vi "Flatten.vi"(6 "Persistence in":refnum<class "IPersist.lvclass">, 7 "Linked List Ref":refnum<data-value>, 8 "error in (no error)":errorcluster, 9 "Indent":i32, 10 "Active Unique ID":string, 11 "Subsequence in":refnum<class "Subsequence.lvclass">) -> (0 "error out":errorcluster, 2 "Active Unique ID out":string, 3 "Flattened Test Executive":string[](array[string]), 4 "Persistence out":refnum<class "IPersist.lvclass">, 5 "Linked List Ref out":refnum<data-value>)   [LabVIEW 2019, in "Test Executive.lvlib" / "Subsequence.lvclass"]
uses:
  <vilib>/gpm_packages/@cs/test-executive/Source/Test Executive/Subsequence/Subsequence.lvclass
  <vilib>/gpm_packages/@cs/linked-list/Source/Linked List/ILinkedList/ILinked List.lvclass
  <vilib>/gpm_packages/@cs/persistence/source/IPersist/IPersist.lvclass
  <vilib>/gpm_packages/@cs/test-executive/Source/Test Executive/Executioner/Executioner.lvclass
  <vilib>/gpm_packages/@cs/linked-list/Source/Linked List/Linked List Ref/Linked List Ref.lvclass
  <vilib>/gpm_packages/@cs/linked-list/Source/String Manipulation/String Manipulation.lvlib
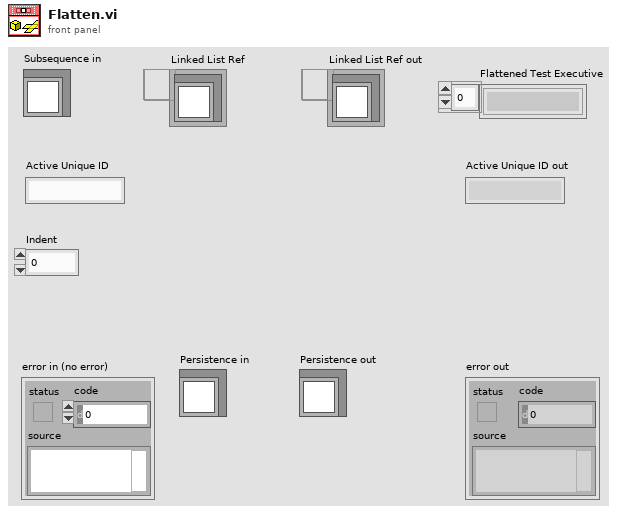
[diagram p1: front panel]
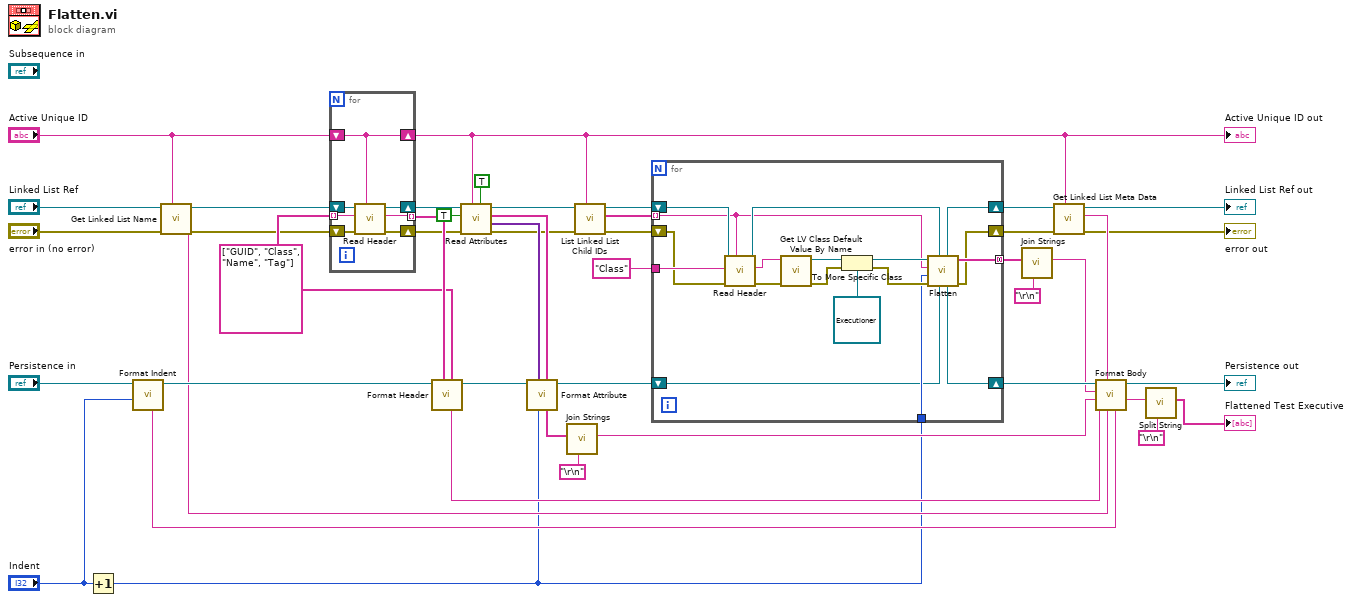
[diagram p0: block diagram]
diagram:
  w37 = string[] ["GUID", "Class", "Name", "Tag"] ("Header Names")
  n1 = Increment(x="Indent") -> (x+1=w17:i32)
  n2 = call-dynamic "Format Indent.vi"("Indent"="Indent", "IPersist in"="Persistence in") -> ("IPersist out"=w41:refnum<class "IPersist.lvclass">, "Indent XML"=w34:string)  [unwired: 7 in, 1 out]
  n3 = call <vilib>:"Get Linked List Name.vi"("Linked List ID"="Active Unique ID", "error in (no error)"="error in (no error)", "Linked List Ref"="Linked List Ref") -> ("error out"=w21:errorcluster, "Linked List Name"=w33:string, "Linked List Ref out"=w44:refnum<data-value>)  [unwired: 5 in, 1 out]
  n4 = for {
    tunnel: w37 -> [w50] mode=indexing
    shift-right: [w51] -> w43
    shift-left: w44 -> [w52]
    tunnel: [w49] -> w38 mode=indexing
    shift-right: [w48] -> w7
    shift-left: "Active Unique ID" -> [w48]
    shift-right: [w46] -> w20
    shift-left: w21 -> [w47]
    n5 = call <vilib>:"Read Header.vi"("Linked List ID"=w48, "error in (no error)"=w47, "Header Name"=w50, "Linked List Ref"=w52) -> ("error out"=w46:errorcluster, "Header Value"=w49:string, "Linked List Ref out"=w51:refnum<data-value>)  [unwired: 4 in, 1 out]
  }
  "Active Unique ID out" <- w7
  n6 = call-dynamic "Format Header.vi"("Name"=w37, "Value"=w38, "IPersist in"=w41) -> ("IPersist out"=w28:refnum<class "IPersist.lvclass">, "Header"=w32:string)  [unwired: 7 in]
  n7 = call <vilib>:"Read Attributes.vi"("Flatten Pointer?"=TRUE, "Linked List ID"=w7, "error in (no error)"=w20, "Include Private?"=TRUE, "Linked List Ref"=w43) -> ("error out"=w19:errorcluster, "Attributes"=w30:variant[], "Attribute Names out"=w29:string[], "Linked List Ref out"=w36:refnum<data-value>)  [unwired: 1 in, 2 out]
  n8 = call-dynamic "Format Attribute.vi"("Attribute Names"=w29, "Indent"=w17, "Attribute Values"=w30, "IPersist in"=w28) -> ("IPersist out"=w16:refnum<class "IPersist.lvclass">, "Attr Strings"=w26:string[])  [unwired: 6 in]
  n9 = call <vilib>:"Join Strings.vi"("Separator (,)"="\r\n", "Strings In"=w26) -> ("String"=w25:string)  [unwired: 9 in]
  n10 = call <vilib>:"List Linked List Child IDs.vi"("Linked List ID"=w7, "error in (no error)"=w19, "Linked List Ref"=w36) -> ("error out"=w4:errorcluster, "Child IDs"=w18:string[], "Linked List Ref out"=w23:refnum<data-value>)  [unwired: 6 in]
  n11 = for {
    shift-right: [w70] -> w22
    shift-left: w23 -> [w69]
    tunnel: w18 -> [w57] mode=indexing
    tunnel: w17 -> [w60]
    shift-right: [w58] -> w15
    shift-left: w16 -> [w59]
    tunnel: [w56] -> w13 mode=concatenating
    shift-right: [w53] -> w2
    shift-left: w4 -> [w54]
    tunnel: "Class" ("Header Name") -> [w55]
    n12 = call <vilib>:"Read Header.vi"("Linked List ID"=w57, "error in (no error)"=w54, "Header Name"=w55, "Linked List Ref"=w69) -> ("error out"=w63:errorcluster, "Header Value"=w64:string, "Linked List Ref out"=w68:refnum<data-value>)  [unwired: 4 in, 1 out]
    n13 = call <vilib>:"Get LV Class Default Value By Name.vi"("error in (no error)"=w63, "class name"=w64) -> ("error out"=w65:errorcluster, "object"=w67:refnum<class>)  [unwired: 8 in]
    n14 = To More Specific Class(target class=refnum<class "Executioner.lvclass"> refnum ("Test Executive.lvlib:Executioner.lvclass"), reference=w67, error in=w65) -> (specific class reference=w62:refnum<class "Executioner.lvclass">, error out=w61:errorcluster)
    n15 = call-dynamic "Flatten.vi"("Persistence in"=w59, "Linked List Ref"=w68, "error in (no error)"=w61, "Indent"=w60, "Active Unique ID"=w57, "Executioner in"=w62) -> ("error out"=w53:errorcluster, "Flattened Test Executive"=w56:string[], "Persistence out"=w58:refnum<class "IPersist.lvclass">, "Linked List Ref out"=w70:refnum<data-value>)  [unwired: 1 in, 1 out]
  }
  n16 = call <vilib>:"Join Strings.vi"("Separator (,)"="\r\n", "Strings In"=w13) -> ("String"=w12:string)  [unwired: 9 in]
  n17 = call <vilib>:"Get Linked List Meta Data.vi"("Linked List ID"=w7, "error in (no error)"=w2, "Linked List Ref"=w22) -> ("error out"=→"error out":errorcluster, "Meta Data"=w24:string, "Linked List Ref out"=→"Linked List Ref out":refnum<data-value>)  [unwired: 5 in, 1 out]
  n18 = call-dynamic "Format Body.vi"("Indent"=w34, "Name"=w33, "Meta Data"=w24, "Header"=w32, "Attributes"=w25, "Body"=w12, "IPersist in"=w15) -> ("String out"=w10:string, "IPersist out"=→"Persistence out":refnum<class "IPersist.lvclass">)  [unwired: 3 in]
  n19 = call <vilib>:"Split String.vi"("Split Pattern"="\r\n", "Input String"=w10) -> ("Split String"=→"Flattened Test Executive":string[])  [unwired: 9 in]
